vi "Register (async).vi"(0 "WAMP Client in":refnum<class "WAMP Client.lvclass">, 1 "Options":string, 5 "Procedure URI":string, 7 "INVOCATION event":refnum<user-event>, 9 "REGISTERED or ERROR event":refnum<user-event>, 11 "error in (no error)":errorcluster) -> (4 "WAMP Client out":refnum<class "WAMP Client.lvclass">, 15 "error out":errorcluster)   [LabVIEW 2020, in "wamplv.lvlib" / "WAMP Client.lvclass"]
uses:
  <vilib>/samangh/wamplv/WAMP Client/WAMP Client.lvclass
  <vilib>/samangh/wamplv/WAMP Client/TypeDef/Success or error.ctl
  <vilib>/samangh/wamplv/WAMP Client/TypeDef/Combined error.ctl
  <vilib>/samangh/wamplv/WAMP Client/TypeDef/WAMP Error Payload.ctl
  <vilib>/samangh/wamplv/WAMP Client/TypeDef/INVOCATION payload.ctl
  <vilib>/samangh/wamplv/WAMP Client/TypeDef/REGISTER Request Data.ctl
  <vilib>/samangh/wamplv/WAMP Client/TypeDef/Internal Message Type.ctl
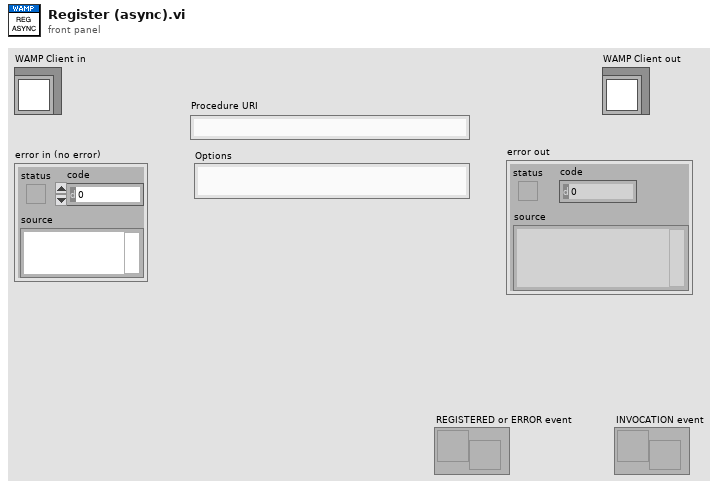
[diagram p1: front panel]
types:
  T1 = typedef "wamplv.lvlib/WAMP Client.lvclass/Internal Message Type.ctl" = enum16{"Subscribe", "Handle Subscribed", "Handle Event", "Unsubscribe", "Handle Unsubscribed", "Publish", "Handled Published", "Goodbye", "Handle Goodbye", "Call", "Handle Result", "Register", "Handle Registered", "Unregister", "Handle Unregistered", "Handle Invocation", "Yield", "Error"}
  T2 = typedef "wamplv.lvlib/WAMP Client.lvclass/REGISTER Request Data.ctl" = cluster{"Procedure URI":string, "Options":string, "REGISTERED or ERROR event":refnum<user-event>, "INVOCATION event":refnum<user-event>}
  T3 = typedef "wamplv.lvlib/WAMP Client.lvclass/Success or error.ctl" = cluster{"Success?":bool, "URI":string, "Combined Error":T4}
  T4 = typedef "wamplv.lvlib/WAMP Client.lvclass/Combined error.ctl" = cluster{"Error?":bool, "WAMP Error":T5, "Error":errorcluster}
  T5 = typedef "wamplv.lvlib/WAMP Client.lvclass/WAMP Error Payload.ctl" = cluster{"Details":string, "ArgumentKw Payload":string, "Wamp error?":bool, "Error URI":string, "Arguments Payload":string[]}
  T6 = typedef "wamplv.lvlib/WAMP Client.lvclass/INVOCATION payload.ctl" = cluster{"Arguments":string[], "ArgumentKw":string, "Procedure URI":string, "Details":string, "Registration ID":u64, "Request ID":u64}
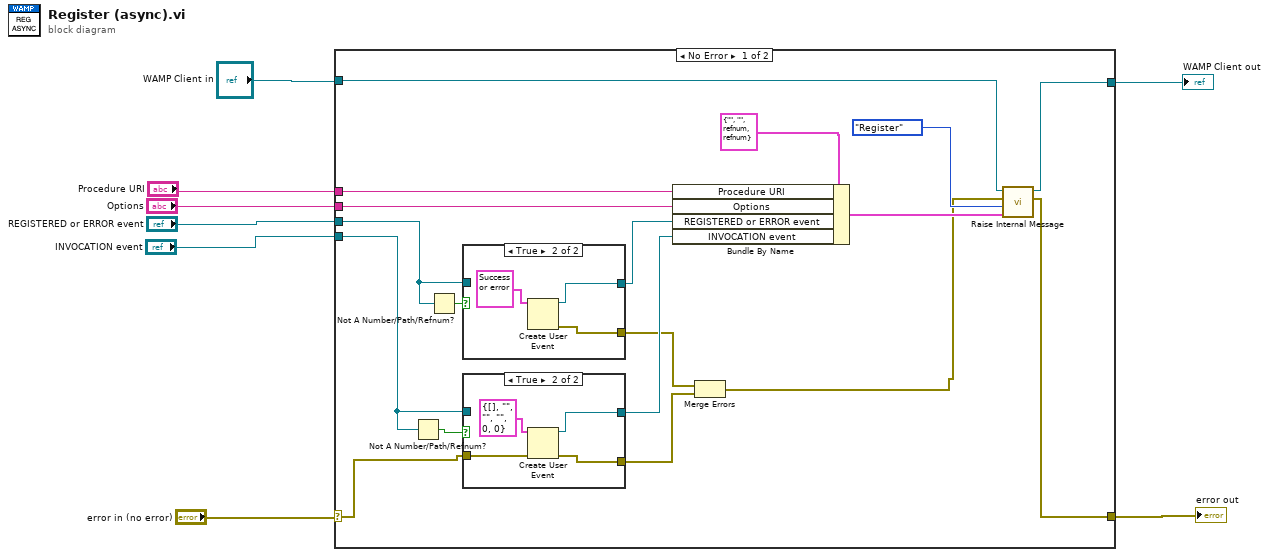
[diagram p0: block diagram]
diagram:
  n1 = case shown="No Error" "error in (no error)" {
    selector: "error in (no error)" -> [w14 w38]
    tunnel: [w19 w38] -> w7
    tunnel: [w22 w37] -> w5
    tunnel: "WAMP Client in" -> [w23 w37]
    tunnel: "Procedure URI" -> [w25 _]
    tunnel: "Options" -> [w24 _]
    tunnel: "REGISTERED or ERROR event" -> [w9 _]
    tunnel: "INVOCATION event" -> [w16 _]
    frame No Error {
      n2 = Not A Number/Path/Refnum?(number/path/refnum=w16) -> (NaN/Path/Refnum?=w18:bool)
      n3 = Not A Number/Path/Refnum?(number/path/refnum=w9) -> (NaN/Path/Refnum?=w10:bool)
      n4 = case shown="True" w10 {
        tunnel: w9 -> [w27 _]
        tunnel: [w27 w30] -> w15
        tunnel: [_ w29] -> w13
        frame False {
        }
        frame True {
          n5 = Create User Event(user event datatype=T3 {"Success?"=FALSE, "URI"="", "Combined Error"={"Error?"=FALSE, "WAMP Error"={"Details"="{}", "ArgumentKw Payload"="", "Wamp error?"=FALSE, "Error URI"="", "Arguments Payload"=[]}, "Error"={"status"=FALSE, "code"=0, "source"=""}}} ("REGISTERED or ERROR payload")) -> (user event=w30:refnum<user-event>, error out=w29:errorcluster)  [unwired: 1 in]
        }
      }
      n6 = case shown="True" w18 {
        tunnel: w16 -> [w32 _]
        tunnel: [w32 w36] -> w17
        tunnel: w14 -> [w31 w34]
        tunnel: [w31 w33] -> w12
        frame False {
        }
        frame True {
          n7 = Create User Event(user event datatype=T6 {"Arguments"=[], "ArgumentKw"="", "Procedure URI"="", "Details"="", "Registration ID"=0, "Request ID"=0} ("INVOCATION payload"), error in=w34) -> (user event=w36:refnum<user-event>, error out=w33:errorcluster)
        }
      }
      n8 = Bundle By Name(cluster=T2 {"Procedure URI"="", "Options"="", "REGISTERED or ERROR event"=refnum, "INVOCATION event"=refnum} ("REGISTER request data"), "Procedure URI"=w25, "Options"=w24, "REGISTERED or ERROR event"=w15, "INVOCATION event"=w17) -> (w20:T2)
      n9 = Merge Errors(w13, w12) -> (w11:errorcluster)
      n10 = call-dynamic "Raise Internal Message.vi"("Variant"=w20, "Internal Message Type"=Internal_Message_Type."Register", "error in (no error)"=w11, "WAMP Client in"=w23) -> ("error out"=w19:errorcluster, "WAMP Client out"=w22:refnum<class "WAMP Client.lvclass">)  [unwired: 6 in]
    }
    frame Error {
    }
  }
  "error out" <- w7
  "WAMP Client out" <- w5
